vi "CreateNewObstacles.vi"(10 "Obstacle Arrays Cluster IN":T1 {"Readable Obstacles"."Obstacle Array"."North" format="%#_10f"; "Readable Obstacles"."Obstacle Array"."East" format="%#_8f"}, 11 "Points of Interest":T3[](array[typedef]) {"North" format="%#_10f"; "East" format="%#_8f"}) -> (2 "Obstacle Arrays Cluster OUT":T1 {"Readable Obstacles"."Obstacle Array"."North" format="%#_10f"; "Readable Obstacles"."Obstacle Array"."East" format="%#_8f"}, 3 "New Obstacle OUT":refnum<class "Obstacle.lvclass">)   [LabVIEW 2013]
doc: "This VI takes in the indicated Mission type and necessary parameters, then creates the Mission object and adds it to\n1) The human readable mission array and\n2) The actual array of mission objects\n\nEric Schneider, August 2014"
uses:
  cRIO_Code/Data/TypeDefs/UTM Location.ctl
  TypeDef/obstacle_arrays.ctl
  cRIO_Code/Logic/Classes/Obstacle/Obstacle.lvclass
  cRIO_Code/Data/TypeDefs/ObstacleDescription.ctl
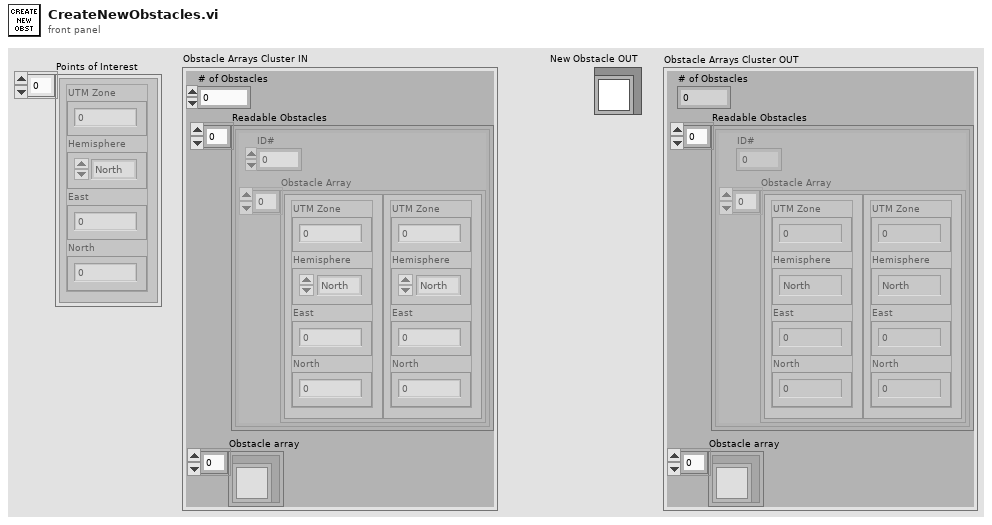
[diagram p1: front panel]
types:
  T1 = typedef "obstacle_arrays.ctl" = cluster{"# of Obstacles":i32, "Obstacle array":refnum<class "Obstacle.lvclass">[], "Readable Obstacles":T2[]}
  T2 = typedef "ObstacleDescription.ctl" = cluster{"ID#":i32, "Obstacle Array":T3[]}
  T3 = typedef "UTM Location.ctl" = cluster{"UTM Zone":dbl, "Hemisphere":enum16{"North", "South"}, "East":dbl, "North":dbl}
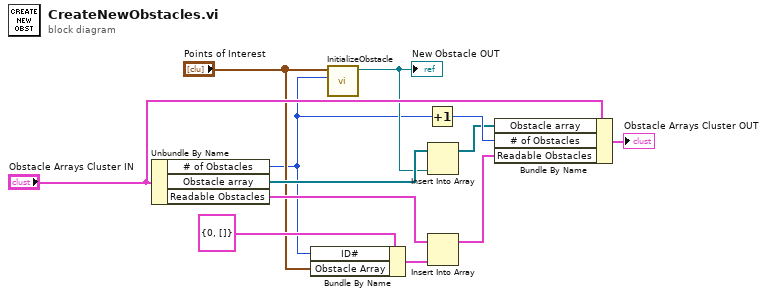
[diagram p0: block diagram]
diagram:
  n1 = Unbundle By Name("Obstacle Arrays Cluster IN") -> ("# of Obstacles"=w1:i32, "Obstacle array"=w11:refnum<class "Obstacle.lvclass">[], "Readable Obstacles"=w10:T2[])
  n2 = Bundle By Name(cluster=T2 {"ID#"=0, "Obstacle Array"=[]} ("Human Readable Obstacle Cluster"), "ID#"=w1, "Obstacle Array"="Points of Interest") -> (w12:T2)
  n3 = call "InitializeObstacle.vi"("ID#"=w1, "Input List of UTM locations to be arranged into segments"="Points of Interest") -> ("Obstacle.lvclass"=w3:refnum<class "Obstacle.lvclass">)  [unwired: 9 in]
  "New Obstacle OUT" <- w3
  n4 = Increment(x=w1) -> (x+1=w8:i32)
  n5 = Insert Into Array(array=w11, new element=w3) -> (w7:refnum<class "Obstacle.lvclass">[])  [unwired: 1 in]
  n6 = Insert Into Array(array=w10, new element=w12) -> (w9:T2[])  [unwired: 1 in]
  n7 = Bundle By Name(cluster="Obstacle Arrays Cluster IN", "Obstacle array"=w7, "# of Obstacles"=w8, "Readable Obstacles"=w9) -> (→"Obstacle Arrays Cluster OUT":T1)
